vi "GetAudioVideoFilenames.vi"(8 "error in (no error)":errorcluster, 9 "Overwrite mode":T1(ring), 10 "Video Filename":string, 11 "Write directory":path) -> (0 "error out":errorcluster, 3 "Video file path":path)   [LabVIEW 2017]
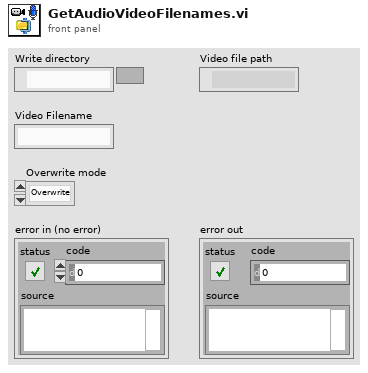
[diagram p1: front panel]
types:
  T1 = enum16{"Overwrite", "Append number", "Append date & time"}
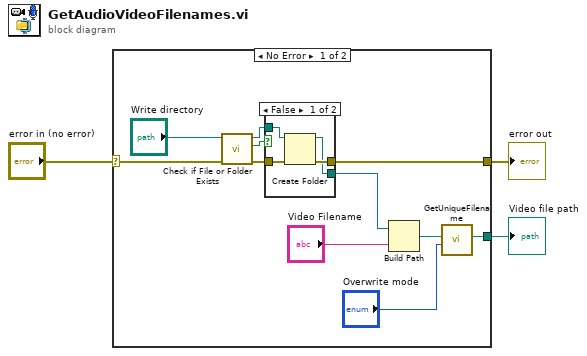
[diagram p0: block diagram]
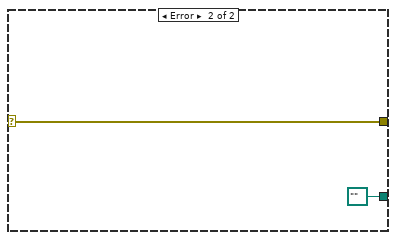
[diagram p3: hidden frame]
diagram:
  n1 = case shown="No Error" "error in (no error)" {
    selector: "error in (no error)" -> [w4 w22]
    tunnel: [w14 w22] -> w3
    tunnel: [w13 path "" ("Output path")] -> w2
    frame No Error {
      n2 = call <vilib>:"Check if File or Folder Exists.vi"("error in (no error)"=w4, "path"="Write directory") -> ("error out"=w8:errorcluster, "file or folder exists?"=w6:bool, "dup path"=w7:path)  [unwired: 7 in]
      n3 = case shown="False" w6 {
        tunnel: w7 -> [w18 w20]
        tunnel: w8 -> [w17 w19]
        tunnel: [w16 w19] -> w14
        tunnel: [w15 w20] -> w9
        frame False {
          n4 = Create Folder(path (use dialog)=w18, error in=w17) -> (created path=w15:path, error out=w16:errorcluster)  [unwired: 1 in, 1 out]
        }
        frame True {
        }
      }
      n5 = Build Path(base path=w9, name or relative path="Video Filename") -> (appended path=w11:path)
      n6 = call "GetUniqueFilename.vi"("Enum"="Overwrite mode", "Input path"=w11) -> ("Output path"=w13:path)  [unwired: 9 in]
    }
    frame Error {
    }
  }
  "error out" <- w3
  "Video file path" <- w2
